vi "SetNegLimit.vi"(0 "Axis In":T1, 5 "Negative Limit":dbl, 11 "error in (no error)":errorcluster) -> (4 "Axis Out":T1, 15 "error out":errorcluster)   [LabVIEW 2009]
doc: "Sets negative software position limit on axis."
uses:
  typedefs/AxisSelect_Enum.ctl
  typedefs/Ultra3000/Cmds.ctl
  typedefs/Ultra3000/Func.ctl
  globals/AxisSpace.vi
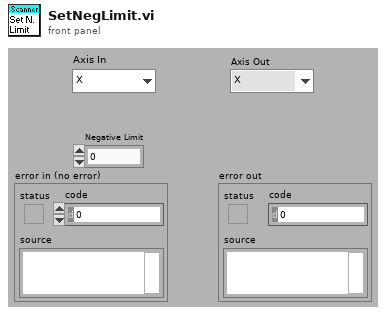
[diagram p1: front panel]
types:
  T1 = typedef "AxisSelect_Enum.ctl" = enum16{"X", "Y", "Z", "Axis Space"}
  T2 = typedef "Func.ctl" = u16
  T3 = typedef "Cmds.ctl" = u16
  T4 = typedef "AxisSpaceCfg.ctl" = T5[]
  T5 = typedef "AxisCfg.ctl" = cluster{"Addr":u8, "Conv Factor":dbl, "Forward Limit":dbl, "Reverse Limit":dbl, "Enable Limits":bool}
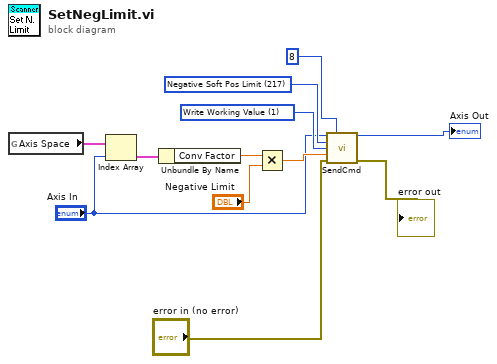
[diagram p0: block diagram]
diagram:
  w11 = T2 1 items=["Read Working Value", "Write Working Value", "Read Non-Volatile Value", "Write Non-Volatile and Woring Value", "Copy Non-Volatile Value to Working Value", "Copy Working Value to Non-Volatile Value", "Read Default Value", "Copy Default Value to Non-Volatile and Working Values", "Read Min Value", "Read Max Value", "Read Array Index Min", "Read Array Index Max"] ("Function")
  w5 = T3 217 items=["Power-Up Status"=1, "Drive Name"=6, "Position Window Size"=22, "Position Window Time"=23, "Zero SPeed Limit"=34, "Speed Window Size"=35, "Up to Speed Limit"=37, "Forward Current Limit"=47, "Reverse Current Limit"=48, "Override Mode"=67, "Operation Mode"=90, "Host Control Mode"=97, "Reset Drive"=106, "Drive Enable"=107, "Setpoint Current"=108, "Setpoint Velocity"=109, "Setpoint Acceleration"=110, "Reset Faults"=111, "Position Comparator"=349, "Postition Comparator Polarity"=350, "Position Rollover Enable"=404, "Baud Rate"=80, "Frame Format"=81, "Drive Address"=82, "Broadcast Address"=83, "Auto-start Indexing"=88, "Start Index"=112, "Host Index"=184, "Index Type"=174, "Index Dist/Pos"=175, "Index Reg Dist"=176, "Index Velocity"=177, "Index Acceleration"=178, "Index Deceleration"=179, "Index Dwell"=180, "Index Count"=181, "Index Termination"=182, "Index Pointer"=183, "Index Abort Deceleration"=185, "Positive Soft Pos Limit"=216, "Negative Soft Pos Limit"=217] ("Command")
  n1 = global read "AxisSpace.vi" "Axis Space"() -> (w10:T4)
  n2 = Index Array(array=w10, index="Axis In") -> (element=w9:T5)
  n3 = Unbundle By Name(w9) -> ("Conv Factor"=w8:dbl)
  n4 = Multiply(x=w8, y="Negative Limit") -> (x*y=w6:dbl)
  n5 = call "SendCmd.vi"("Axis In"="Axis In", "Data Length Constant (0)"=u8 8 ("DLC"), "Command"=w5, "Function"=w11, "Data (0)"=w6, "error in (no error)"="error in (no error)") -> ("Axis Out"=→"Axis Out":T1, "error out"=→"error out":errorcluster)  [unwired: 6 in, 2 out]
